vi "Dispose Image Refs.vi"(1 "error in (no error)":errorcluster, 2 "Image Refs":T1) -> (0 "error out":errorcluster)   [LabVIEW 2020]
uses:
  Type Defs/Image Refs.ctl
  <vilib>/vision/Image Controls.llb/IMAQ Image.ctl
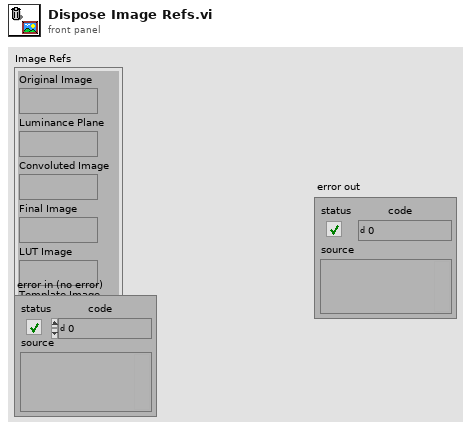
[diagram p1: front panel]
types:
  T1 = typedef "Image Refs.ctl" = cluster{"Original Image":T2, "Luminance Plane":T2, "Convoluted Image":T2, "Final Image":T2, "LUT Image":T2, "Template Image":T2}
  T2 = typedef "IMAQ Image.ctl" = refnum<image>
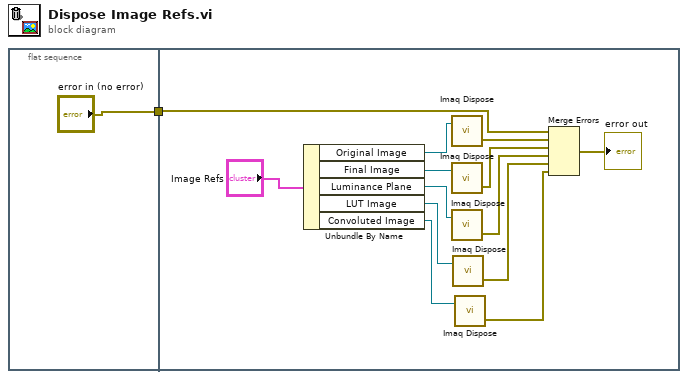
[diagram p0: block diagram]
diagram:
  n1 = flat-sequence {
    tunnel: ["error in (no error)"] -> w1
    tunnel: w1 -> [w5]
    frame #0 {
    }
    frame #1 {
      n2 = Unbundle By Name("Image Refs") -> ("Original Image"=w12:T2, "Final Image"=w13:T2, "Luminance Plane"=w14:T2, "LUT Image"=w8:T2, "Convoluted Image"=w4:T2)
      n3 = call "Imaq Dispose"("Image"=w12) -> ("error out"=w11:errorcluster)  [unwired: 5 in]
      n4 = call "Imaq Dispose"("Image"=w13) -> ("error out"=w10:errorcluster)  [unwired: 5 in]
      n5 = call "Imaq Dispose"("Image"=w14) -> ("error out"=w9:errorcluster)  [unwired: 5 in]
      n6 = call "Imaq Dispose"("Image"=w8) -> ("error out"=w7:errorcluster)  [unwired: 5 in]
      n7 = call "Imaq Dispose"("Image"=w4) -> ("error out"=w3:errorcluster)  [unwired: 5 in]
      n8 = Merge Errors(w5, w11, w10, w9, w7, w3) -> (→"error out":errorcluster)
    }
  }
